vi "Read analogue FIFO data.vi"(11 "?":T1) -> (0 "error out":errorcluster, 1 "Data read":bool, 2 "Data":sgl[](array[numeric]), 3 "?":T1)   [LabVIEW 2018]
uses:
  Type Defs/Analogue loop data.ctl
  Type Defs/FPGA reference.ctl
  <vilib>/Utility/error.llb/Error Cluster From Error Code.vi
  <vilib>/rvi/errors/niLvFpgaAdjustHostInterfaceError.vi
  <vilib>/rvi/interface/nirviMethod/nirviMethod.xnode
  FPGA Bitfiles/CompressorRigV2_CompressorFPGA_FPGAMainV3_7sPRekuravM.lvbitx
  <vilib>/rvi/errors/niLvFpgaMergeErrorWithErrorCode.vi
  <vilib>/FPGAPlugInAG/cRIO-9056/niLvFpga_ReadFifo_cRIO-9056.vi
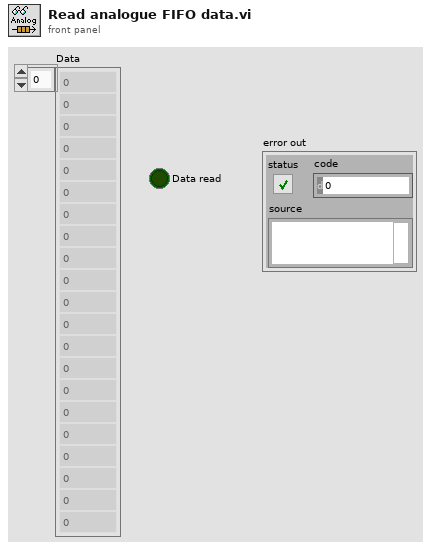
[diagram p1: front panel]
types:
  T1 = typedef "Analogue loop data.ctl" = cluster{"Params":cluster{"FPGA ref":T2, "Total Channels":u32}, "Variables":cluster{"FIFO wait counter":u16, "FIFO read trigger":u32}}
  T2 = typedef "FPGA reference.ctl" = refnum<k20>
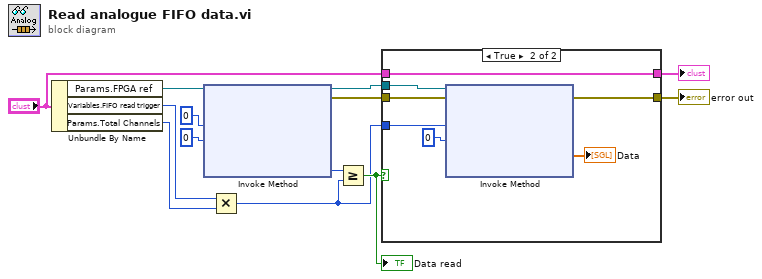
[diagram p0: block diagram]
diagram:
  n1 = Unbundle By Name("?") -> ("Params.FPGA ref"=w10:T2, "Variables.FIFO read trigger"=w2:u32, "Params.Total Channels"=w3:u32)
  n2 = xnode "Invoke Method"("FPGA VI Reference In"=w10, "Number of Elements"=u32 0, "Timeout (ms)"=0) -> ("FPGA VI Reference Out"=w1:T2, "error out"=w6:errorcluster, "Elements Remaining"=w7:u32)  [unwired: 1 in, 1 out]
  n3 = Multiply(x=w2, y=w3) -> (x*y=w4:u32)
  n4 = Greater Or Equal?(x=w7, y=w4) -> (x >= y?=w11:bool)
  "Data read" <- w11
  n5 = case shown="True" w11 {
    tunnel: w1 -> [_ w22]
    tunnel: w4 -> [_ w21]
    tunnel: "?" -> [w14 w16]
    tunnel: [w14 w16] -> w9
    tunnel: w6 -> [w15 w19]
    tunnel: [w15 w18] -> w5
    frame False {
    }
    frame True {
      n6 = xnode "Invoke Method"("FPGA VI Reference In"=w22, "error in"=w19, "Number of Elements"=w21, "Timeout (ms)"=0) -> ("error out"=w18:errorcluster, "Data"=→"Data":sgl[])  [unwired: 2 out]
    }
  }
  "?" <- w9
  "error out" <- w5
